vi "ImplModelFollow_Calculate.vi"(9 "U":T1, 10 "X":T1, 11 "in IMPLICIT_MODEL_FOLLOWER":T2) -> (0 "Error":bool, 2 "U Out":T1, 3 "out IMPLICIT_MODEL_FOLLOWER":T2)   [LabVIEW 2019, in "Trajectory_Library.lvlib"]
doc: "Create implicit model follower\n\nInputs:\n - A < states, states > -- Continuous system matrix of the plant being controlled.\n - B < states, inputs > -- Continuous input matrix of the plant being controlled.\n - A_Ref < states, states > -- Continuous system matrix whose dymanics should be followed.\n - B_Ref < states, inputs > -- Continuous input matrix x whose dymanics should be followed.\n\nOutputs:\n - Error -- If TRUE, an error occured."
uses:
  Trajectory_Library.lvlib
  TypeDef/IMPLICIT_MODEL_FOLLOWER.ctl
  <vilib>/Analysis/Matrix/Datatypes/RealMatrix.ctl
  <vilib>/Analysis/baseanly.llb/Real A x B.vi
  <vilib>/Analysis/Matrix/Numeric/Add/Add - RM,RM.vi
  <vilib>/Analysis/NI_AALBase.lvlib
  <vilib>/Analysis/Matrix/NI_Matrix.lvlib
panel:
  # "<Inputs, 1>"
  # "<States, 1>"
  # "<Inputs, 1>"
  # "<States,States>"
  # "<States,Inputs>"
  # "<Inputs,1>"
  # "<States,States>"
  # "<States,Inputs>"
  # "<Inputs,1>"
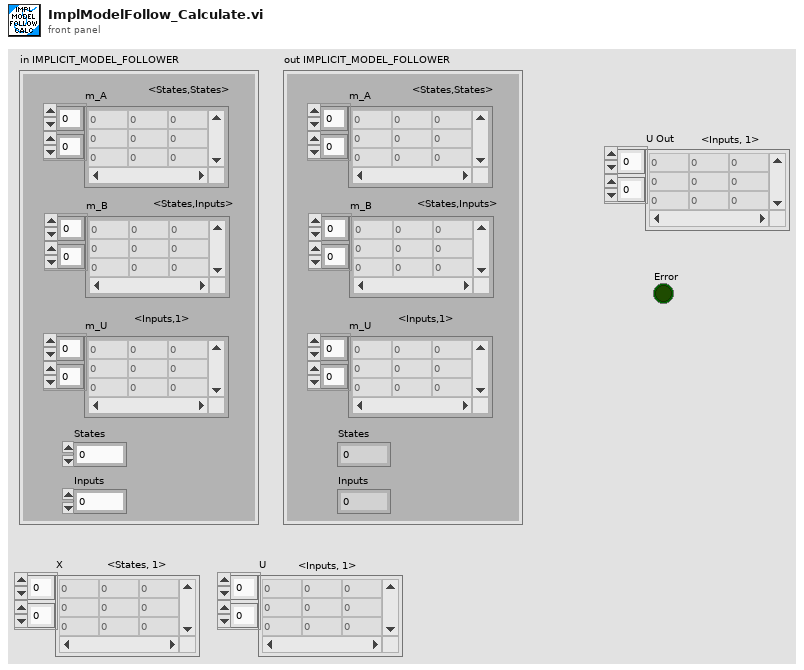
[diagram p1: front panel]
types:
  T1 = typedef "NI_Matrix.lvlib/RealMatrix.ctl" = dbl[][]
  T2 = typedef "Trajectory_Library.lvlib/IMPLICIT_MODEL_FOLLOWER.ctl" = cluster{"m_A":T1, "m_B":T1, "m_U":T1, "States":i32, "Inputs":i32}
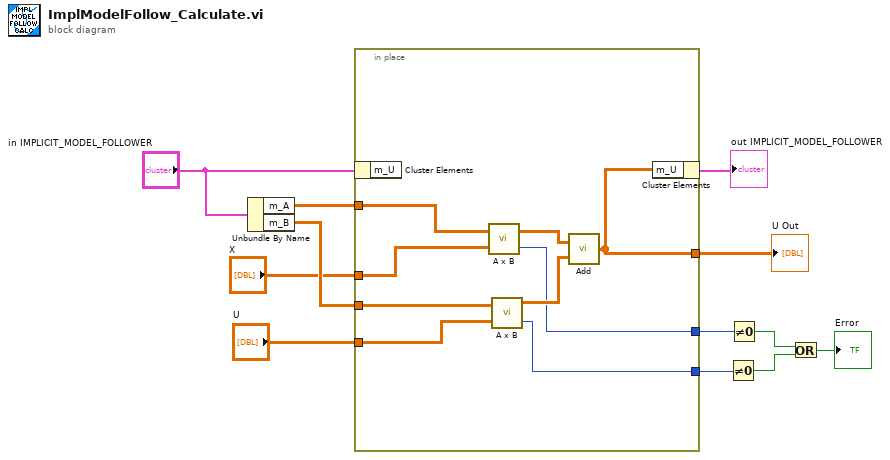
[diagram p0: block diagram]
diagram:
  n1 = Unbundle By Name("in IMPLICIT_MODEL_FOLLOWER") -> ("m_A"=w10:T1, "m_B"=w9:T1)
  n2 = in-place {
    in-place-border: w10 -> [w21]
    in-place-border: w9 -> [w20]
    in-place-border: "X" -> [w19]
    in-place-border: "U" -> [w18]
    in-place-border: [w15] -> w6
    in-place-border: [w14] -> w3
    in-place-border: [w13] -> w2
    n3 = in-place-cluster #1("in IMPLICIT_MODEL_FOLLOWER") -> ()  [unwired: 1 out]
    n4 = call-poly <vilib>:"A x B.vi"("B"=w19, "A"=w21) -> ("error"=w14:i32, "A x B"=w17:T1)
    n5 = call-poly <vilib>:"A x B.vi"("B"=w18, "A"=w20) -> ("error"=w13:i32, "A x B"=w16:T1)
    n6 = call-poly <vilib>:"Add.vi"("Real Matrix B"=w16, "Real Matrix A"=w17) -> ("A + B"=w15:T1)
    n7 = in-place-cluster #1("m_U"=w15) -> (→"out IMPLICIT_MODEL_FOLLOWER":T2)
  }
  "U Out" <- w6
  n8 = Not Equal To 0?(x=w2) -> (x != 0?=w4:bool)
  n9 = Not Equal To 0?(x=w3) -> (x != 0?=w5:bool)
  n10 = Or(x=w5, y=w4) -> (x .or. y?=→"Error":bool)
